vi "LatchSetLinkState.vi"(10 "LatchLinkState":bool) -> ()   [LabVIEW 2014, in "LatchLib.lvlib"]
uses:
  LatchLib.lvlib
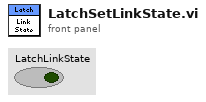
[diagram p1: front panel]
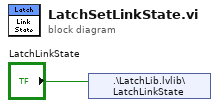
[diagram p0: block diagram]
diagram:
  n1 = shared-variable ".\\LatchLib.lvlib\\LatchLinkState"("LatchLinkState") -> ()  [unwired: 1 in, 1 out]
